vi "Actor Core.vi"(8 "error in":errorcluster, 11 "Nested in":refnum<class "C100L.lvclass">) -> (0 "error out":errorcluster, 3 "Actor out":refnum<class "Actor.lvclass">)   [LabVIEW 2021, in "C100L.lvlib" / "C100L.lvclass"]
doc: "(<B>Filename</B>: Actor Framework.lvlib:Actor.lvclass:Actor Core.vi)\n\nReceives messages to the actor, reacts to them, and initiates any error handling that may shut the actor down.\n\nDescendant classes may override this VI to append parallel tasks for the actor to complete while it handles messages. Overrides use the Call Parent Method node."
uses:
  C100L.lvclass
  C100L.lvclass/C100L.ctl
  <vilib>/ActorFramework/Actor/Actor.lvclass
  <vilib>/ActorFramework/Stop Msg/Stop Msg.lvclass
  C100L Messages/Upd Flow Setpoint Msg/Upd Flow Setpoint Msg.lvclass
  C100L Messages/Upd Desired Gas Msg/Upd Desired Gas Msg.lvclass
  C100L Messages/Upd Full Scale Range Msg/Upd Full Scale Range Msg.lvclass
  <vilib>/MGI/Panel Manager/Panel Actor/Panel Actor/Panel Actor.lvclass
  C100L Messages/Upd MFC Calibrated Gas Msg/Upd MFC Calibrated Gas Msg.lvclass
  C:/Program Files/National Instruments/LabVIEW 2021/vi.lib/ActorFramework/Actor/Actor.lvclass
panel:
  in  "Full Scale Range":dbl
  in  "Desired Gas":string(combo)
  in  "MFC Calibrated Gas":string(combo)
  in  "Flow Setpoint":dbl(slide) scale=0.0..10.0
  out "Flow Measured":dbl(slide) scale=0.0..10.0
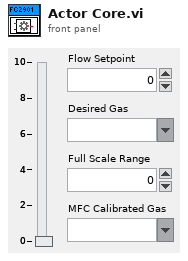
[diagram p1: front panel]
types:
  T1 = cluster{"Stop":refnum<user-event>, "Flow Measured":refnum<user-event>}
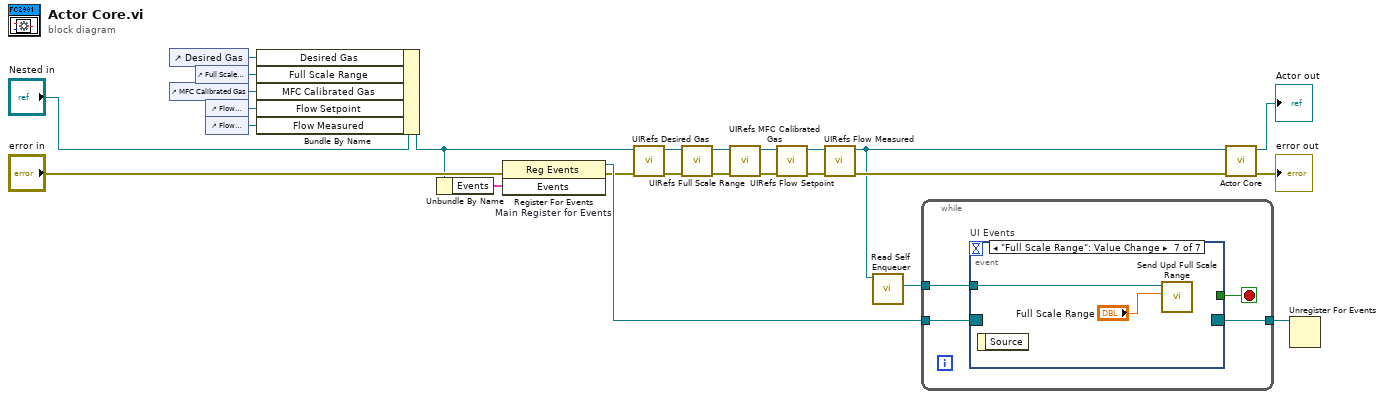
[diagram p0: block diagram]
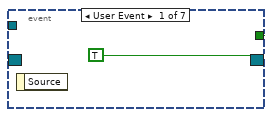
[diagram p2: hidden frame]
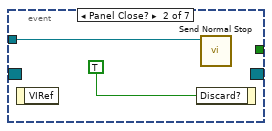
[diagram p3: hidden frame]
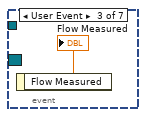
[diagram p4: hidden frame]
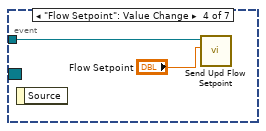
[diagram p5: hidden frame]
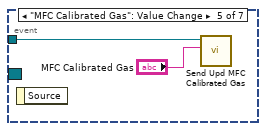
[diagram p6: hidden frame]
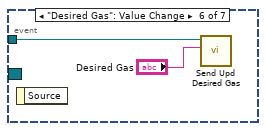
[diagram p7: hidden frame]
diagram:
  n1 = control-ref of="Desired Gas"() -> (w1:refnum<vi>)
  n2 = control-ref of="MFC Calibrated Gas"() -> (w3:refnum<vi>)
  n3 = control-ref of="Full Scale Range"() -> (w2:refnum<vi>)
  n4 = control-ref of="Flow Setpoint"() -> (w4:refnum<vi>)
  n5 = control-ref of="Flow Measured"() -> (w5:refnum<vi>)
  n6 = Bundle By Name(cluster="Nested in", "Desired Gas"=w1, "Full Scale Range"=w2, "MFC Calibrated Gas"=w3, "Flow Setpoint"=w4, "Flow Measured"=w5) -> (w9:refnum<class "C100L.lvclass">)
  n7 = Unbundle By Name(w9) -> ("Events"=w22:T1)
  n8 = register-events "Main Register for Events"(error in="error in", w22) -> (reference out=w23:refnum<event-registration>, error out=w8:errorcluster)  [unwired: 1 in]
  n9 = call "UIRefs Desired Gas.vi"("error in (no error)"=w8, "C100L in"=w9) -> ("error out"=w7:errorcluster, "C100L out"=w6:refnum<class "C100L.lvclass">)  [unwired: 8 in]
  n10 = call "UIRefs Full Scale Range.vi"("error in (no error)"=w7, "C100L in"=w6) -> ("error out"=w16:errorcluster, "C100L out"=w17:refnum<class "C100L.lvclass">)  [unwired: 8 in]
  n11 = call "UIRefs MFC Calibrated Gas.vi"("error in (no error)"=w16, "C100L in"=w17) -> ("error out"=w10:errorcluster, "C100L out"=w11:refnum<class "C100L.lvclass">)  [unwired: 8 in]
  n12 = call "UIRefs Flow Setpoint.vi"("error in (no error)"=w10, "C100L in"=w11) -> ("error out"=w15:errorcluster, "C100L out"=w13:refnum<class "C100L.lvclass">)  [unwired: 8 in]
  n13 = call "UIRefs Flow Measured.vi"("error in (no error)"=w15, "C100L in"=w13) -> ("error out"=w14:errorcluster, "C100L out"=w12:refnum<class "C100L.lvclass">)  [unwired: 8 in]
  n14 = call <vilib>:"Read Self Enqueuer.vi"("Actor"=w12) -> ("Self Enqueuer"=w20:refnum<class "Message Enqueuer.lvclass">)  [unwired: 10 in]
  n15 = while {
    tunnel: w23 -> [w29]
    tunnel: [w27] -> w21
    tunnel: w20 -> [w26]
    stop <- w28 stop-if-true
    n16 = event "UI Events" shown="[6] \"Full Scale Range\": Value Change" {
      selector: w29 -> [_ _ _ _ _ _ _]
      dyn-events: [_ _ _ _ _ _ _] -> w27
      timeout: _ -> [_ _ _ _ _ _ _]
      tunnel: [TRUE _ _ _ _ _ _] -> w28
      tunnel: w26 -> [_ w31 _ w35 w37 w39 w41]
      event User Event {
        n17 = event-data() -> ()  [unwired: 1 in, 1 out]
      }
      event Panel Close? {
        n18 = event-data() -> ()  [unwired: 1 in, 1 out]
        n19 = event-data("Discard?"=TRUE) -> ()  [unwired: 1 in, 1 out]
        n20 = call <vilib>:"Send Normal Stop.vi"("Message Enqueuer"=w31) -> ()  [unwired: 10 in, 1 out]
      }
      event User Event {
        n21 = event-data() -> ("Flow Measured"=→"Flow Measured":dbl)  [unwired: 1 in]
      }
      event "Flow Setpoint": Value Change {
        n22 = event-data() -> ()  [unwired: 1 in, 1 out]
        n23 = call "Send Upd Flow Setpoint.vi"("Flow Setpoint"="Flow Setpoint", "Message Enqueuer"=w35) -> ()  [unwired: 8 in, 2 out]
      }
      event "MFC Calibrated Gas": Value Change {
        n24 = event-data() -> ()  [unwired: 1 in, 1 out]
        n25 = call "Send Upd MFC Calibrated Gas.vi"("MFC Calibrated Gas"="MFC Calibrated Gas", "Message Enqueuer"=w37) -> ()  [unwired: 8 in, 2 out]
      }
      event "Desired Gas": Value Change {
        n26 = event-data() -> ()  [unwired: 1 in, 1 out]
        n27 = call "Send Upd Desired Gas.vi"("Desired Gas"="Desired Gas", "Message Enqueuer"=w39) -> ()  [unwired: 8 in, 2 out]
      }
      event "Full Scale Range": Value Change {
        n28 = event-data() -> ()  [unwired: 1 in, 1 out]
        n29 = call "Send Upd Full Scale Range.vi"("Full Scale Range"="Full Scale Range", "Message Enqueuer"=w41) -> ()  [unwired: 8 in, 2 out]
      }
    }
  }
  n30 = call-parent "Actor Core.vi"("error in"=w14, "Panel Actor in"=w12) -> ("error out"=→"error out":errorcluster, "Actor out"=→"Actor out":refnum<class "Actor.lvclass">)  [unwired: 8 in]
  n31 = Unregister For Events(event registration refnum=w21) -> ()  [unwired: 1 in, 1 out]
